vi "DI4_Scope.vi"() -> ()   [LabVIEW 2015, in "ECS-Host.lvlib"]
uses:
  ECS-Host.lvlib
panel:
  out "DI4_Scope":sgl[][](graph)
  in  "DI4_ScopeRefresh":bool
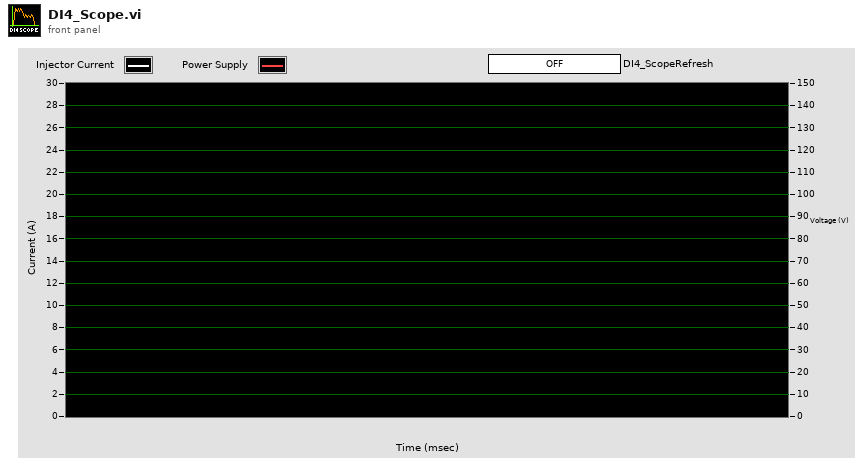
[diagram p1: front panel]
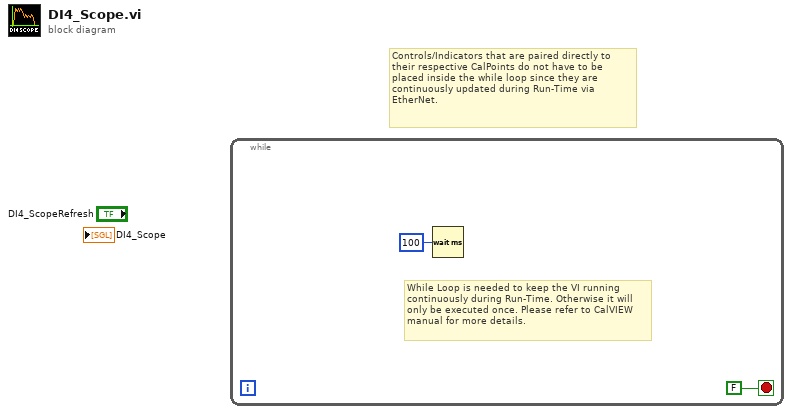
[diagram p0: block diagram]
diagram:
  # "Controls/Indicators that are paired directly to their respective CalPoints do not have to be placed inside the while loop since they are continuously updated during Run-Time via EtherNet."
  n1 = while {
    stop <- FALSE stop-if-true
    # "While Loop is needed to keep the VI running\ncontinuously during Run-Time. Otherwise it will only be executed once. Please refer to CalVIEW manual for more details."
    n2 = Wait (ms)(milliseconds to wait=u32 100) -> ()  [unwired: 1 out]
  }
